vi "chipKIT Secondary UART.vi"() -> ()   [LabVIEW 2011, in "LabVIEW Interface for ChipKit.lvlib"]
uses:
  vi.lib/LabVIEW Interface for ChipKit/LabVIEW Interface for ChipKit.lvlib
panel:
  in  "Data":string
  in  "Buad Rate":u32=9600
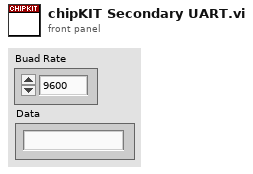
[diagram p1: front panel]
types:
  T1 = typedef "LabVIEW Interface for ChipKit.lvlib/Chipkit Resource.ctl" = cluster{"COM Port":refnum<visa-resource-name>, "Board Type":T2, "Connection Type":T3, "Baud Rate (115200)":u32, "Bytes Per Packet (15)":u32}
  T2 = typedef "LabVIEW Interface for ChipKit.lvlib/Board Type.ctl" = enum16{"ChipKit uC32", "ChipKit Uno32", "ChipKit Max32"}
  T3 = typedef "LabVIEW Interface for ChipKit.lvlib/Connection Type.ctl" = enum8{"USB / Serial", "XBEE", "BlueSmirf (Bluetooth)"}
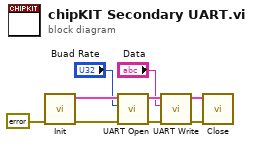
[diagram p0: block diagram]
diagram:
  n1 = call "Init.vi"("Error In"=errorcluster {"status"=FALSE, "code"=0, "source"=""}) -> ("Error Out"=w4:errorcluster, "ChipKit Configuration"=w9:T1)  [unwired: 9 in]
  n2 = call "UART Open.vi"("Error In"=w4, "Buad Rate"="Buad Rate", "ChipKit Resource 2"=w9) -> ("Error Out"=w5:errorcluster, "ChipKit Resource"=w8:T1)  [unwired: 7 in]
  n3 = call "UART Write.vi"("Error In"=w5, "Data"="Data", "ChipKit Resource 2"=w8) -> ("Error Out"=w6:errorcluster, "ChipKit Resource"=w7:T1)  [unwired: 7 in]
  n4 = call "Close.vi"("Error In"=w6, "ChipKit Configuration"=w7) -> ()  [unwired: 9 in, 1 out]
